vi "全局变量.vi"() -> ()   [LabVIEW 2018]
panel:
  out "悬停":dbl
  out "定向":dbl
  out "定深":dbl
  out "启动模式":dbl
  out "速度档位":dbl
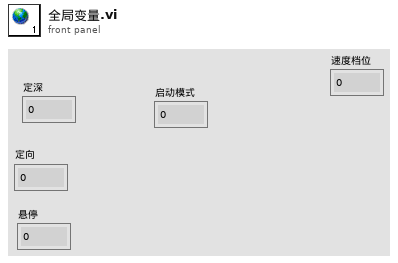
[diagram p1: front panel]
diagram:
